vi "Value_JSON.vi"(0 "Data JSON":string, 5 "Type":string, 7 "Size data":string, 9 "Hexa":string, 11 "error in":errorcluster) -> (4 "Value_string":string, 8 "Hexa value":string, 15 "error IO":errorcluster)   [LabVIEW 2021]
uses:
  <vilib>/JDP Science/JSONtext/String Subset.vi
  <vilib>/JDP Science/JSONtext/support/Strip Quotes and Unescape.vi
  <vilib>/JDP Science/JSONtext/support/Unescape JSON string.vi
  <vilib>/JDP Science/JSONtext/Parsing/Parse Full Path or Item Name.vi
  <vilib>/JDP Science/JSONtext/Offset/Find Item Locations by Path.vi
  <vilib>/JDP Science/JSONtext/JSONtext.lvlib
panel:
  out "Data JSON 2":string
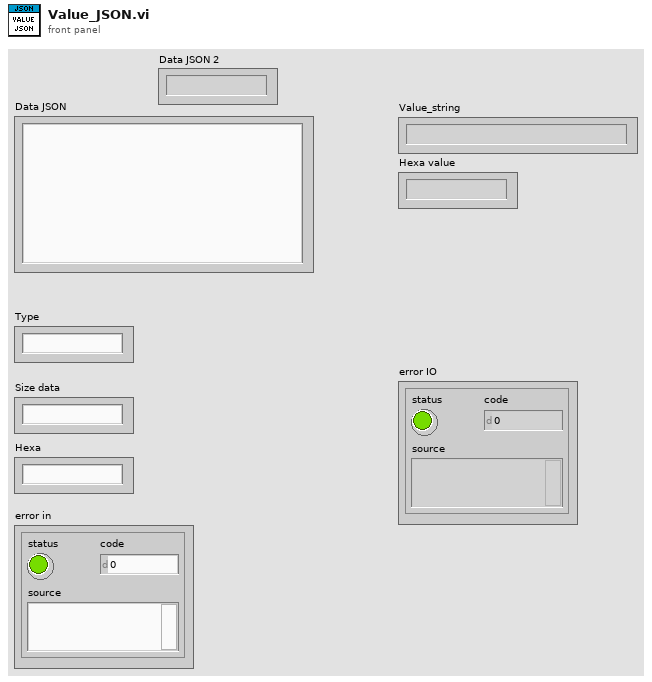
[diagram p1: front panel]
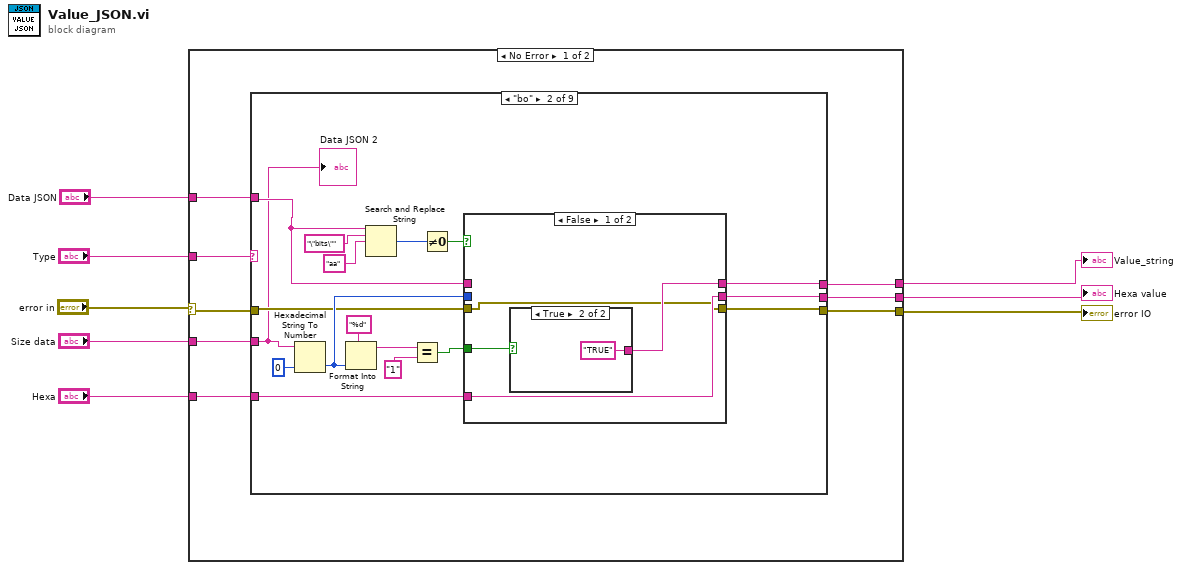
[diagram p0: block diagram]
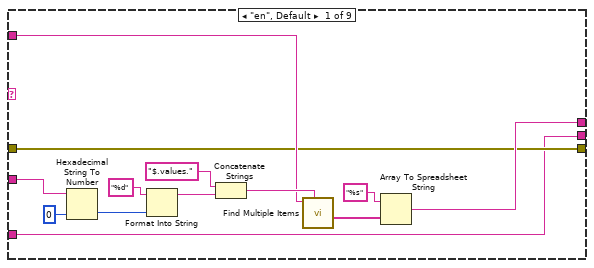
[diagram p2: hidden frame]
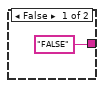
[diagram p3: hidden frame]
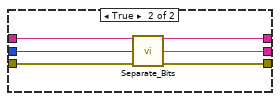
[diagram p4: hidden frame]
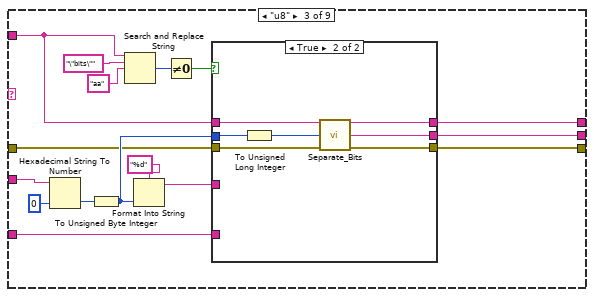
[diagram p5: hidden frame]
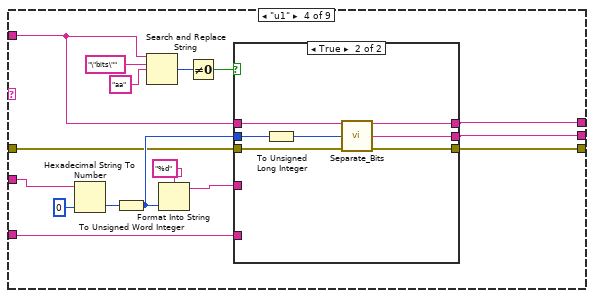
[diagram p7: hidden frame]
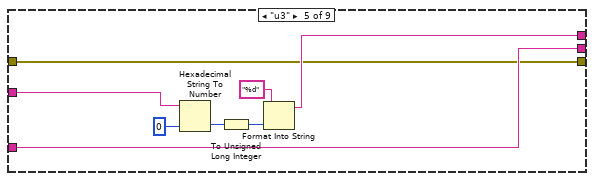
[diagram p9: hidden frame]
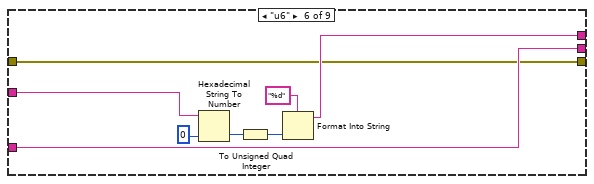
[diagram p10: hidden frame]
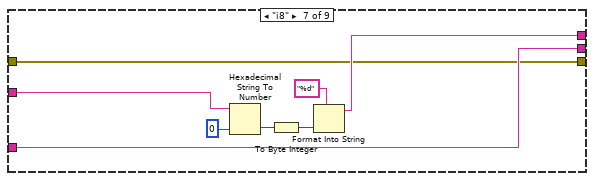
[diagram p11: hidden frame]
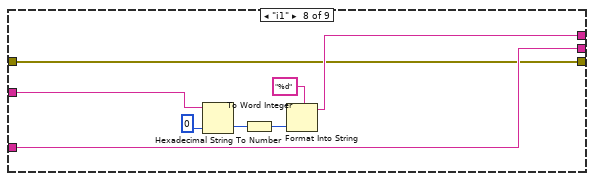
[diagram p12: hidden frame]
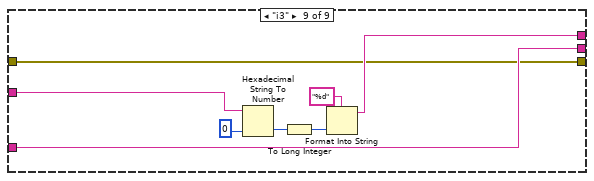
[diagram p13: hidden frame]
diagram:
  n1 = case shown="No Error" "error in" {
    selector: "error in" -> [w13 w151]
    tunnel: "Data JSON" -> [w16 _]
    tunnel: "Size data" -> [w15 _]
    tunnel: "Type" -> [w9 _]
    tunnel: "Hexa" -> [w14 _]
    tunnel: [w12 w151] -> w2
    tunnel: [w11 _] -> w3
    tunnel: [w10 _] -> w1
    frame No Error {
      n2 = case shown="\"bo\"" w9 {
        tunnel: w15 -> [w23 w30 w67 w90 w114 w122 w130 w138 w146]
        tunnel: [w20 w38 w65 w88 w113 w121 w129 w137 w145] -> w10
        tunnel: [w17 w37 w62 w87 w112 w120 w128 w136 w144] -> w11
        tunnel: w14 -> [w17 w36 w63 w91 w112 w120 w128 w136 w144]
        tunnel: w16 -> [w19 w31 w64 w89 _ _ _ _ _]
        tunnel: w13 -> [w18 w34 w60 w86 w111 w119 w127 w135 w143]
        tunnel: [w18 w33 w59 w85 w111 w119 w127 w135 w143] -> w12
        frame "en", Default {
          n3 = Hexadecimal String To Number(string=w23, default (0uL)=u32 0 ("default (0 U32)")) -> (number=w29:u32)  [unwired: 1 in, 1 out]
          n4 = Format Into String(format string="%d", w29) -> (resulting string=w26:string)  [unwired: 2 in, 1 out]
          n5 = Concatenate Strings("$.values." ("string"), w26) -> (w25:string)
          n6 = call <vilib>:"Find Multiple Items.vi"("$Path or Item Name"=w25, "JSON"=w19) -> ("<JSON>"=w21:string[])  [unwired: 6 in, 3 out]
          n7 = Array To Spreadsheet String(array=w21, 3:"%s" ("format string")) -> (spreadsheet string=w20:string)  [unwired: 1 in]
        }
        frame "bo" {
          n8 = Hexadecimal String To Number(string=w30, default (0uL)=u32 0 ("default (0 U32)")) -> (number=w35:u32)  [unwired: 1 in, 1 out]
          n9 = Format Into String(format string="%d", w35) -> (resulting string=w45:string)  [unwired: 2 in, 1 out]
          n10 = Search and Replace String(input string=w31, search string="\"bits\"", replace string="aa" ("replace string (\"\")")) -> (number of replacements=w40:i32)  [unwired: 5 in, 3 out]
          n11 = Equal?(x=w45, y="1") -> (x = y?=w39:bool)
          n12 = Not Equal To 0?(x=w40) -> (x != 0?=w32:bool)
          n13 = case shown="False" w32 {
            tunnel: [w49 w56] -> w38
            tunnel: w31 -> [_ w58]
            tunnel: [w48 w55] -> w37
            tunnel: w39 -> [w50 _]
            tunnel: w36 -> [w48 _]
            tunnel: w35 -> [_ w57]
            tunnel: w34 -> [w47 w54]
            tunnel: [w47 w53] -> w33
            frame False {
              n14 = case shown="True" w50 {
                tunnel: ["FALSE" "TRUE"] -> w49
                frame False {
                }
                frame True {
                }
              }
            }
            frame True {
              n15 = call "Separate_Bits.vi"("JSON"=w58, "int size number"=w57, "error in"=w54) -> ("Value_string"=w56:string, "hex_data"=w55:string, "error out"=w53:errorcluster)  [unwired: 10 in]
            }
          }
          "Data JSON 2" <- w30
        }
        frame "u8" {
          n16 = Hexadecimal String To Number(string=w67, default (0uL)=u32 0 ("default (0 U32)")) -> (number=w72:u32)  [unwired: 1 in, 1 out]
          n17 = To Unsigned Byte Integer(number=w72) -> (unsigned 8bit integer=w61:u8)
          n18 = Search and Replace String(input string=w64, search string="\"bits\"", replace string="aa" ("replace string (\"\")")) -> (number of replacements=w69:i32)  [unwired: 5 in, 3 out]
          n19 = Format Into String(format string="%d", w61) -> (resulting string=w66:string)  [unwired: 2 in, 1 out]
          n20 = Not Equal To 0?(x=w69) -> (x != 0?=w68:bool)
          n21 = case shown="True" w68 {
            tunnel: [w77 w81] -> w65
            tunnel: w66 -> [w77 _]
            tunnel: w64 -> [_ w84]
            tunnel: w63 -> [w76 _]
            tunnel: [w76 w80] -> w62
            tunnel: w61 -> [_ w83]
            tunnel: w60 -> [w75 w79]
            tunnel: [w75 w78] -> w59
            frame False {
            }
            frame True {
              n22 = To Unsigned Long Integer(number=w83) -> (unsigned 32bit integer=w82:u32)
              n23 = call "Separate_Bits.vi"("JSON"=w84, "int size number"=w82, "error in"=w79) -> ("Value_string"=w81:string, "hex_data"=w80:string, "error out"=w78:errorcluster)  [unwired: 10 in]
            }
          }
        }
        frame "u1" {
          n24 = Hexadecimal String To Number(string=w90, default (0uL)=u32 0 ("default (0 U32)")) -> (number=w96:u32)  [unwired: 1 in, 1 out]
          n25 = To Unsigned Word Integer(number=w96) -> (unsigned 16bit integer=w100:u16)
          n26 = Search and Replace String(input string=w89, search string="\"bits\"", replace string="aa" ("replace string (\"\")")) -> (number of replacements=w97:i32)  [unwired: 5 in, 3 out]
          n27 = Format Into String(format string="%d", w100) -> (resulting string=w99:string)  [unwired: 2 in, 1 out]
          n28 = Not Equal To 0?(x=w97) -> (x != 0?=w98:bool)
          n29 = case shown="True" w98 {
            tunnel: [w103 w107] -> w88
            tunnel: w99 -> [w103 _]
            tunnel: w89 -> [_ w110]
            tunnel: w91 -> [w102 _]
            tunnel: [w102 w106] -> w87
            tunnel: w100 -> [_ w109]
            tunnel: w86 -> [w101 w105]
            tunnel: [w101 w104] -> w85
            frame False {
            }
            frame True {
              n30 = To Unsigned Long Integer(number=w109) -> (unsigned 32bit integer=w108:u32)
              n31 = call "Separate_Bits.vi"("JSON"=w110, "int size number"=w108, "error in"=w105) -> ("Value_string"=w107:string, "hex_data"=w106:string, "error out"=w104:errorcluster)  [unwired: 10 in]
            }
          }
        }
        frame "u3" {
          n32 = Hexadecimal String To Number(string=w114, default (0uL)=u32 0 ("default (0 U32)")) -> (number=w117:u32)  [unwired: 1 in, 1 out]
          n33 = To Unsigned Long Integer(number=w117) -> (unsigned 32bit integer=w118:u32)
          n34 = Format Into String(format string="%d", w118) -> (resulting string=w113:string)  [unwired: 2 in, 1 out]
        }
        frame "u6" {
          n35 = Hexadecimal String To Number(string=w122, default (0uL)=u32 0 ("default (0 U32)")) -> (number=w125:u32)  [unwired: 1 in, 1 out]
          n36 = To Unsigned Quad Integer(1:w125) -> (0:w126:u64)
          n37 = Format Into String(format string="%d", w126) -> (resulting string=w121:string)  [unwired: 2 in, 1 out]
        }
        frame "i8" {
          n38 = Hexadecimal String To Number(string=w130, default (0uL)=u32 0 ("default (0 U32)")) -> (number=w133:u32)  [unwired: 1 in, 1 out]
          n39 = To Byte Integer(number=w133) -> (8bit integer=w134:i8)
          n40 = Format Into String(format string="%d", w134) -> (resulting string=w129:string)  [unwired: 2 in, 1 out]
        }
        frame "i1" {
          n41 = Hexadecimal String To Number(string=w138, default (0uL)=u32 0 ("default (0 U32)")) -> (number=w141:u32)  [unwired: 1 in, 1 out]
          n42 = To Word Integer(number=w141) -> (16bit integer=w142:i16)
          n43 = Format Into String(format string="%d", w142) -> (resulting string=w137:string)  [unwired: 2 in, 1 out]
        }
        frame "i3" {
          n44 = Hexadecimal String To Number(string=w146, default (0uL)=u32 0 ("default (0 U32)")) -> (number=w149:u32)  [unwired: 1 in, 1 out]
          n45 = To Long Integer(number=w149) -> (32bit integer=w150:i32)
          n46 = Format Into String(format string="%d", w150) -> (resulting string=w145:string)  [unwired: 2 in, 1 out]
        }
      }
    }
    frame Error {
    }
  }
  "Value_string" <- w1
  "Hexa value" <- w3
  "error IO" <- w2
